vi "get dependency list.vi"(8 "error in":errorcluster, 11 "Shared Library Module editor node in":refnum<class "Shared Library Module editor node.lvclass">) -> (0 "error out":errorcluster, 2 "files":T1[](array[typedef]), 3 "Shared Library Module editor node out":refnum<class "Shared Library Module editor node.lvclass">)   [LabVIEW 2013, in "Shared Library Module editor node.lvclass"]
uses:
  Shared Library Module editor node.lvclass
  <vilib>/NI/DCAF/Tag Editor Core/Configuration Editor/Classes/TBM Configuration Node/deployment configuration.ctl
  <vilib>/NI/DCAF/Tag Editor Core/Configuration Editor/Classes/Module editor node/module editor node.lvclass
  Shared Library Module editor node.lvclass/Shared Library Module editor node.ctl
  configuration/Shared Library Module configuration.lvclass/Shared Library Module configuration.ctl
  Read local path.vi
  <vilib>/NI/DCAF/Tag Editor Core/Configuration Editor/Classes/Module editor node/Write Module Configuration.vi
  <vilib>/NI/Configuration Framework/serializable configuration/read metadata property.vi
  <vilib>/NI/DCAF/Tag Editor Core/Configuration Editor/Classes/Module editor node/Read Module Configuration.vi
  configuration/Shared Library Module configuration.lvclass
  <vilib>/NI/DCAF/Tag Editor Core/Configuration Editor/Classes/TBM Configuration Node/TBM Configuration Node.lvclass
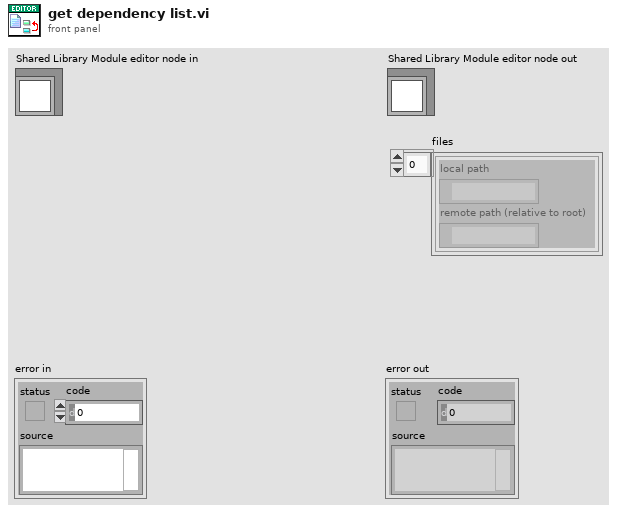
[diagram p1: front panel]
types:
  T1 = typedef "PL Framework Configuration Tool.lvlib/TBM Configuration Node.lvclass/deployment configuration.ctl" = cluster{"local path":path, "remote path (relative to root)":path}
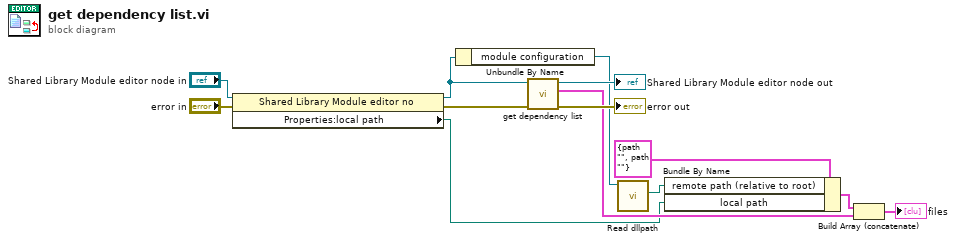
[diagram p0: block diagram]
diagram:
  n1 = property class="Shared Library Module editor no"(reference="Shared Library Module editor node in", error in="error in") -> (reference out=w2:refnum<class "Shared Library Module editor node.lvclass">, error out=w4:errorcluster, "Properties:local path"=w1:path)
  n2 = Unbundle By Name(w2) -> ("module configuration"=w9:refnum<class "Shared Library Module configuration.lvclass">)
  n3 = call-parent "get dependency list.vi"("error in"=w4, "TBM Configuration Node in"=w2) -> ("error out"=→"error out":errorcluster, "files"=w12:T1[], "TBM Configuration Node out"=→"Shared Library Module editor node out":refnum<class "Shared Library Module editor node.lvclass">)  [unwired: 7 in]
  n4 = call "Read dllpath.vi"("Shared Library Module configuration in"=w9) -> ("dllpath"=w6:path)  [unwired: 8 in, 2 out]
  n5 = Bundle By Name(cluster=T1 {"local path"=path "", "remote path (relative to root)"=path ""} ("deployment configuration"), "remote path (relative to root)"=w6, "local path"=w1) -> (w5:T1)
  n6 = Build Array (concatenate)(w5, w12) -> (→"files":T1[])
